vi "Data_Limit.vi"(8 "Error In":errorcluster caption="错误输入", 9 "最小值":dbl, 10 "最大值":dbl, 11 "输入值":dbl) -> (0 "Error Out":errorcluster caption="错误输出", 2 "超出界限":bool, 3 "颜色":u32(colorbox))   [LabVIEW 2020]
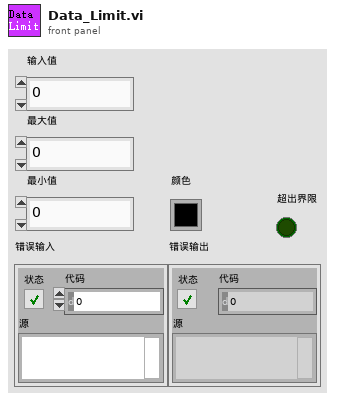
[diagram p1: front panel]
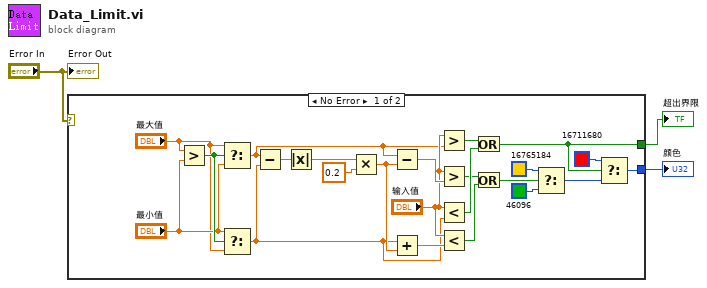
[diagram p0: block diagram]
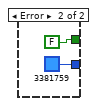
[diagram p2: hidden frame]
diagram:
  n1 = case shown="No Error" "Error In" {
    tunnel: [w23 u32 3381759 ("颜色")] -> w3
    tunnel: [w18 FALSE] -> w1
    frame No Error {
      n2 = Greater?(x="最大值", y="最小值") -> (0:w7:bool)
      n3 = Select(t="最大值", s=w7, f="最小值") -> (s? t:f=w8:dbl)
      n4 = Select(t="最小值", s=w7, f="最大值") -> (s? t:f=w4:dbl)
      n5 = Subtract(x=w8, y=w4) -> (x-y=w17:dbl)
      n6 = Absolute Value(x=w17) -> (abs(x)=w16:dbl)
      n7 = Multiply(x=w16, y=0.2) -> (x*y=w14:dbl)
      n8 = Subtract(x=w8, y=w14) -> (x-y=w13:dbl)
      n9 = Add(x=w4, y=w14) -> (x+y=w11:dbl)
      n10 = Greater?(x="输入值", y=w8) -> (0:w25:bool)
      n11 = Greater?(x="输入值", y=w13) -> (0:w10:bool)
      n12 = Less?(x="输入值", y=w4) -> (x < y?=w26:bool)
      n13 = Less?(x="输入值", y=w11) -> (x < y?=w9:bool)
      n14 = Or(x=w25, y=w26) -> (x .or. y?=w18:bool)
      n15 = Or(x=w10, y=w9) -> (x .or. y?=w22:bool)
      n16 = Select(t=u32 16765184 ("颜色"), s=w22, f=u32 46096 ("颜色")) -> (s? t:f=w19:u32)
      n17 = Select(t=u32 16711680 ("颜色"), s=w18, f=w19) -> (s? t:f=w23:u32)
    }
    frame Error {
    }
  }
  "颜色" <- w3
  "超出界限" <- w1
  "Error Out" <- "Error In"
